vi "PH_uOPA_DelayController.evt call set Sample Length.vi"(0 "i ref in":refnum<vi>, 2 "Instance":string="N/A", 3 "Sample Length":i32, 5 "error in (no error)":errorcluster) -> (14 "i ref out":refnum<vi>, 19 "error out":errorcluster)   [LabVIEW 2014, in "PH_uOPA_DelayController.lvlib"]
doc: "This VI calls the \"GetData\" case."
uses:
  PH_uOPA_DelayController.lvlib
  CS_Core/CSSystem/CoreLib/CoreLib.int 2 byte array.vi
  CS_Core/BaseProcess/BaseProcess.lvlib
  CS_Core/CSSystem/CoreLib/CoreLib.lvlib
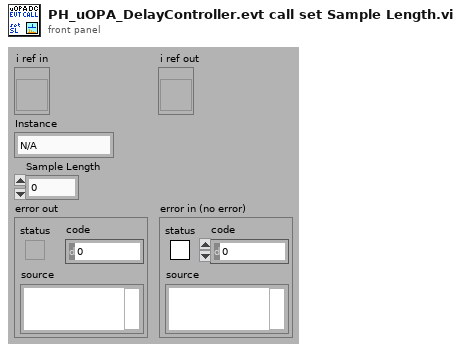
[diagram p1: front panel]
types:
  T1 = typedef "CoreDefs.rawDataType.ctl" = i8[]
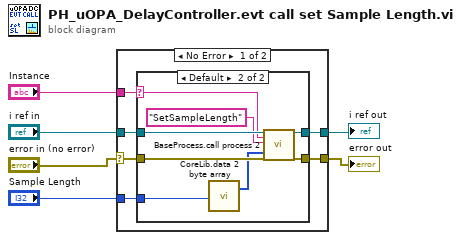
[diagram p0: block diagram]
diagram:
  n1 = case shown="No Error" "error in (no error)" {
    selector: "error in (no error)" -> [w9 w24]
    tunnel: [w12 w23] -> w6
    tunnel: [w11 w24] -> w5
    tunnel: "i ref in" -> [w10 w23]
    tunnel: "Instance" -> [w8 _]
    tunnel: "Sample Length" -> [w7 _]
    frame No Error {
      n2 = case shown="Default" w8 {
        selector: w8 -> [_ w17]
        tunnel: [w14 w22] -> w12
        tunnel: [w13 w21] -> w11
        tunnel: w10 -> [w14 w20]
        tunnel: w9 -> [w13 w18]
        tunnel: w7 -> [_ w15]
        frame "N/A" {
        }
        frame Default {
          n3 = call-poly "CoreLib.data 2 byte array.vi"("i32"=w15) -> ("byteArray out"=w16:T1)  [unwired: 18 in]
          n4 = call "BaseProcess.call process 2.vi"("i ref in"=w20, "Object"=w17, "Selector"="SetSampleLength", "Data"=w16, "error in (no error)"=w18) -> ("i ref out"=w22:refnum<vi>, "error out"=w21:errorcluster)  [unwired: 13 in]
        }
      }
    }
    frame Error {
    }
  }
  "error out" <- w5
  "i ref out" <- w6
